vi "UpdateMatlabExpParameter.vi"(8 "error in (no error)":errorcluster, 9 "Invoke (t)?":bool=TRUE, 10 "Parameter(s)":variant, 11 "ExpID":string) -> (0 "error out":errorcluster)   [LabVIEW 2017]
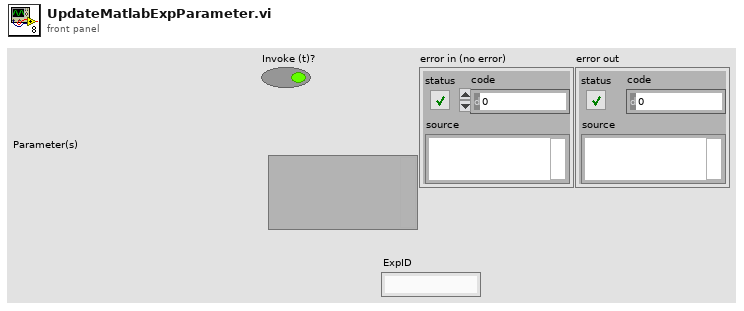
[diagram p1: front panel]
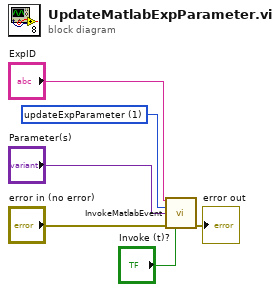
[diagram p0: block diagram]
diagram:
  w5 = u16 1 items=["[FromStringName]", "updateExpParameter", "invokeMethod"] ("Event")
  n1 = call "InvokeMatlabEvent.vi"("ExpID"="ExpID", "Event"=w5, "Data"="Parameter(s)", "error in (no error)"="error in (no error)", "Invoke?"="Invoke (t)?") -> ("error out"=→"error out":errorcluster)  [unwired: 10 in]
